vi "Global 2.vi"() -> ()   [LabVIEW 2020]
panel:
  out "New_M":dbl
  in  "FowardBackward":dbl
  out "TInit":dbl
  out "Measure":bool
  out "Velocity (m/s)":dbl
  out "Z":dbl
  out "Y":dbl
  out "X":dbl
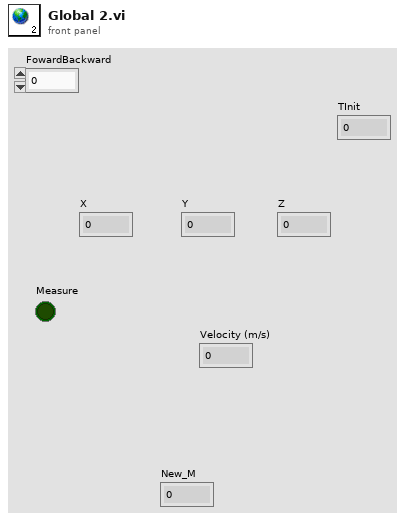
[diagram p1: front panel]
diagram:
